vi "Auto OS index.vi"(1 "Sampling rate":sgl=1000.0) -> (0 "OS index":u8=6)   [LabVIEW 2014]
panel:
  in  "Frequency thresholds (Hz)":sgl[](array[numeric])=[1500.0, 3000.0, 6000.0, 12000.0, 21500.0, 28900.0, 33000.0]
  # ">"
  # "64"
  # ">"
  # "32"
  # ">"
  # "16"
  # ">"
  # "8"
  # ">"
  # "4"
  # ">"
  # "2"
  # ">"
  # "1"
  # "OS ratio"
  # "PN 19/12/2014"
  # "(must be in ascending order)"
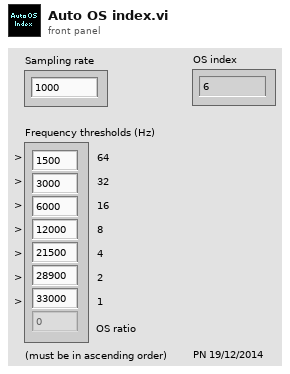
[diagram p1: front panel]
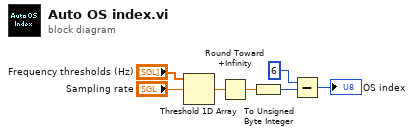
[diagram p0: block diagram]
diagram:
  n1 = Threshold 1D Array(2:"Sampling rate", 3:"Frequency thresholds (Hz)") -> (0:w5:sgl)  [unwired: 1 in]
  n2 = Round Toward +Infinity(x=w5) -> (ceil(x): smallest int >= x=w4:sgl)
  n3 = To Unsigned Byte Integer(number=w4) -> (unsigned 8bit integer=w3:u8)
  n4 = Subtract(x=u8 6, y=w3) -> (x-y=→"OS index":u8)
